vi "QuerySelectionValue.vi"(8 "error in (no error)":errorcluster, 11 "ExcuseNotesHandler in":refnum<class "ExcuseNotesHandler.lvclass">) -> (0 "error out":errorcluster, 3 "ExcuseNotesHandler out":refnum<class "ExcuseNotesHandler.lvclass">)   [LabVIEW 2015, in "Admin_Actor.lvlib" / "ExcuseNotesHandler.lvclass"]
uses:
  ExcuseNotesHandler.lvclass
  ExcuseNotesHandler.lvclass/ExcuseNotesHandler.ctl
  Global Variable/g_Pos_Determine.vi
  ListSelection.lvclass
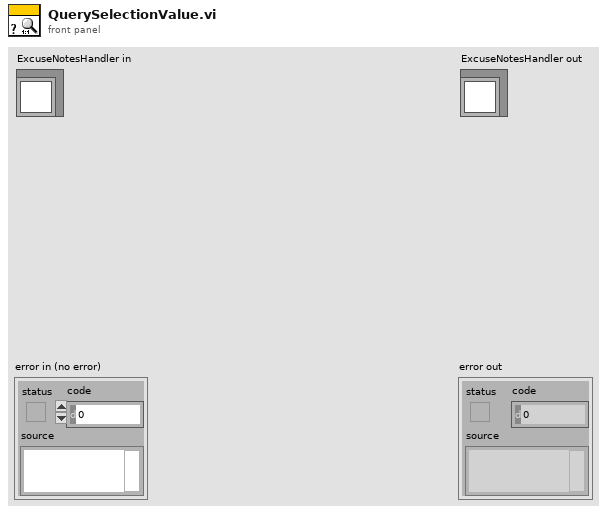
[diagram p1: front panel]
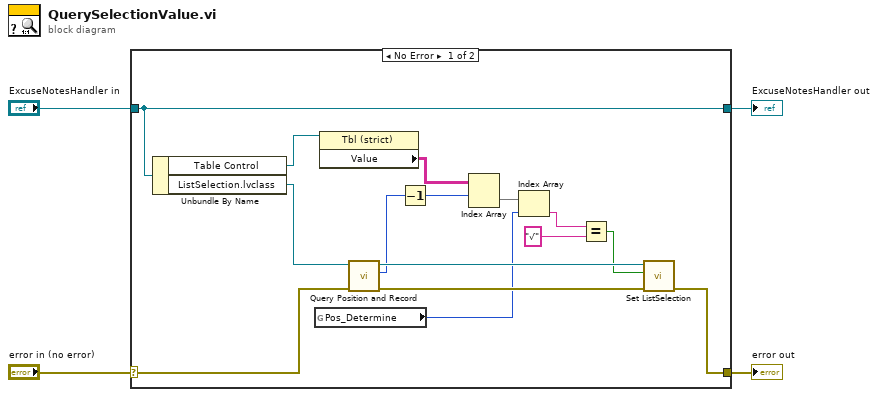
[diagram p0: block diagram]
diagram:
  n1 = case shown="No Error" "error in (no error)" {
    selector: "error in (no error)" -> [w11 w21]
    tunnel: [w8 w21] -> w3
    tunnel: [w19 w20] -> w1
    tunnel: "ExcuseNotesHandler in" -> [w19 w20]
    frame No Error {
      n2 = Unbundle By Name(w19) -> ("Table Control"=w18:refnum<vi>, "ListSelection.lvclass"=w16:refnum<class "ListSelection.lvclass">)
      n3 = global read "g_Pos_Determine.vi" "Pos_Determine"() -> (w7:i32)
      n4 = property class="Tbl (strict)"(reference=w18) -> ("Value"=w17:string[][])  [unwired: 1 in, 2 out]
      n5 = call "Query Position and Record.vi"("error in (no error)"=w11, "ListSelection in"=w16) -> ("error out"=w10:errorcluster, "InxOfColumns"=w6:i32, "ListSelection out"=w12:refnum<class "ListSelection.lvclass">)  [unwired: 6 in, 1 out]
      n6 = Decrement(x=w6) -> (x-1=w5:i32)
      n7 = Index Array(array=w17, index (row)=w5) -> (element=w15:string[])  [unwired: 1 in]
      n8 = Index Array(array=w15, index=w7) -> (element=w14:string)
      n9 = Equal?(x=w14, y="√") -> (x = y?=w9:bool)
      n10 = call "Set ListSelection.vi"("error in (no error)"=w10, "BooelanValue(False)"=w9, "ListSelection in"=w12) -> ("error out"=w8:errorcluster)  [unwired: 7 in, 1 out]
    }
    frame Error {
    }
  }
  "error out" <- w3
  "ExcuseNotesHandler out" <- w1
